vi "Cal_Pos_Max_Min.vi"(0 "Positions":dbl[][](array[numeric]) format="%.2f") -> (1 "Position Info":string[][](array[string]), 2 "Instrument moved?":bool)   [LabVIEW 2010]
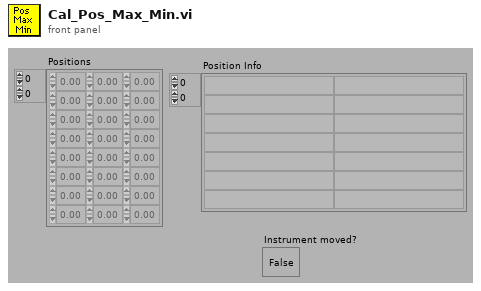
[diagram p1: front panel]
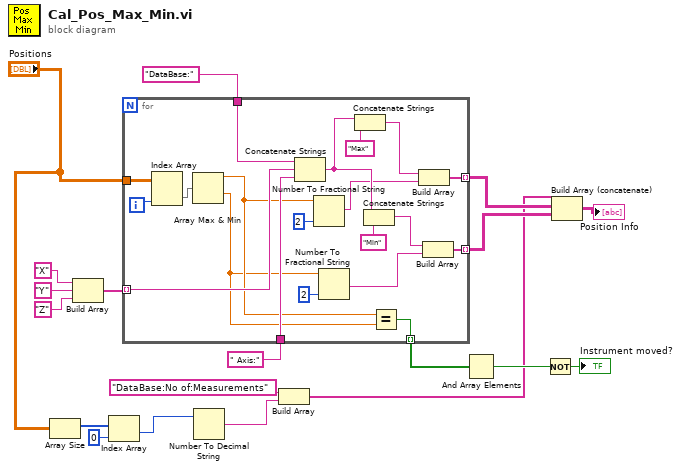
[diagram p0: block diagram]
diagram:
  n1 = Array Size(array="Positions") -> (size(s)=w5:i32[])
  n2 = Build Array("X", "Y", "Z") -> (w14:string[])
  n3 = Index Array(array=w5, index=0) -> (element=w3:i32)
  n4 = for {
    tunnel: "Positions" -> [w39]
    tunnel: "DataBase:" -> [w36]
    tunnel: w14 -> [w35] mode=indexing
    tunnel: " Axis:" -> [w34]
    tunnel: [w24] -> w16 mode=indexing
    tunnel: [w23] -> w17 mode=indexing
    tunnel: [w20] -> w19 mode=indexing
    i -> [w37]
    n5 = Index Array(array=w39, index (col)=w37) -> (element=w38:dbl[])  [unwired: 1 in]
    n6 = Array Max & Min(array=w38) -> (max value=w22:dbl, min value=w21:dbl)  [unwired: 2 out]
    n7 = Concatenate Strings(w36, w35, w34) -> (w30:string)
    n8 = Number To Fractional String(number=w22, precision (6)=i16 2) -> (F-format string=w26:string)  [unwired: 2 out]
    n9 = Number To Fractional String(number=w21, precision (6)=i16 2) -> (F-format string=w25:string)  [unwired: 2 out]
    n10 = Concatenate Strings(w30, "Max") -> (w33:string)
    n11 = Concatenate Strings(w30, "Min") -> (w29:string)
    n12 = Equal?(x=w22, y=w21) -> (x = y?=w20:bool)
    n13 = Build Array(w33, w26) -> (w24:string[])
    n14 = Build Array(w29, w25) -> (w23:string[])
  }
  n15 = Number To Decimal String(number=w3) -> (decimal integer string=w2:string)  [unwired: 1 out]
  n16 = Build Array("DataBase:No of:Measurements", w2) -> (w1:string[])
  n17 = And Array Elements(Boolean array=w19) -> (logical AND=w9:bool)
  n18 = Not(x=w9) -> (.not. x?=→"Instrument moved?":bool)
  n19 = Build Array (concatenate)(w1, w16, w17) -> (→"Position Info":string[][])
